vi "Construct Text Log Sink.vi"(7 "LogLevel":T1, 10 "File Name":string, 11 "Log File Folder":path) -> (3 "Text File Sink out":refnum<class "Text File Sink.lvclass">)   [LabVIEW 2018, in "MVA Framework.lvlib" / "Text File Sink.lvclass"]
doc: "Construct an instance of text log sink. If no file name is input, the file name will be 'Application Directory Name Event Log'. If no log file folder is input, the log file folder will be Public Application Data\\Application Directory Name Event Logs. \n - File extension used is .txt. \n - File will be rolled over at 1Mb.\n - File name will include a timestamp when that file was created.\nFor control over these default values, use the advanced constructor."
uses:
  Text File Sink.lvclass
  Composed Log/Log Sink/Log Sink.lvclass
  Configuration.ctl
  <vilib>/Utility/sysdir.llb/System Directory Type.ctl
  Composed Log/Types/Log Level.ctl
  Composed Log/Composed Log.lvlib
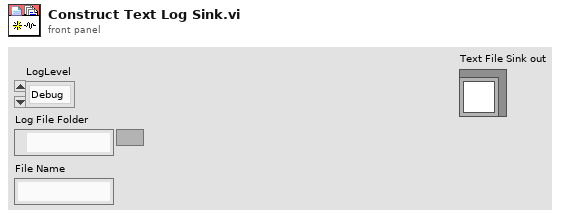
[diagram p1: front panel]
types:
  T1 = typedef "MVA Framework.lvlib/Composed Log.lvlib/Log Level.ctl" = enum16{"Debug", "Info", "Warning", "Error", "Critical"}
  T2 = typedef "MVA Framework.lvlib/Text File Sink.lvclass/Configuration.ctl" = cluster{"Folder":path, "Name":string, "Extension":string, "Max Size (MB)":i64, "Timestamp Filename":bool}
  T3 = typedef "System Directory Type.ctl" = i32
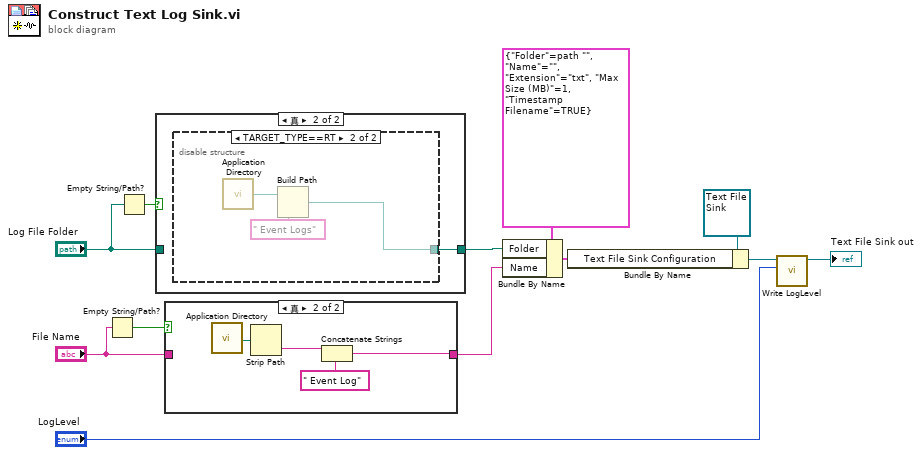
[diagram p0: block diagram]
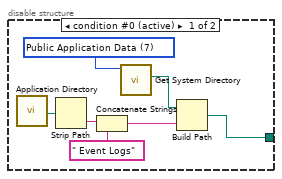
[diagram p4: hidden frame]
diagram:
  n1 = Empty String/Path?(string/path="File Name") -> (empty?=w4:bool)
  n2 = Empty String/Path?(string/path="Log File Folder") -> (empty?=w7:bool)
  n3 = case shown="真" w7 {
    tunnel: "Log File Folder" -> [w13 _]
    tunnel: [w13 w14] -> w5
    frame False {
    }
    frame True {
      n4 = disable-structure shown="TARGET_TYPE==RT" {
        disable-tunnel: [w15 w22] -> w14
        frame condition #0 (active) {
          w21 = T3 7 items=["User Home"=0, "User Desktop"=1, "User Documents"=2, "User Application Data"=3, "User Preferences"=4, "User Temporary"=5, "Public Documents"=6, "Public Application Data"=7, "Public Preferences"=8, "Public Cache"=13, "System Core Libraries"=9, "System Installed Libraries"=10, "Application Files"=11, "Boot Volume Root"=12] ("system directory type")
          n5 = call <vilib>:"Application Directory.vi"() -> ("Application Directory"=w20:path)
          n6 = Strip Path(path=w20) -> (name=w19:string)  [unwired: 1 out]
          n7 = Concatenate Strings(w19, " Event Logs" ("string")) -> (w17:string)
          n8 = call <vilib>:"Get System Directory.vi"("system directory type"=w21) -> ("system directory"=w16:path)  [unwired: 10 in]
          n9 = Build Path(base path=w16, name or relative path=w17) -> (appended path=w15:path)
        }
        frame condition #1 {
          n10 = call <vilib>:"Application Directory.vi"() -> ("Application Directory"=w23:path)
          n11 = Build Path(base path=w23, name or relative path=" Event Logs" ("string")) -> (appended path=w22:path)
        }
      }
    }
  }
  n12 = case shown="真" w4 {
    tunnel: "File Name" -> [w25 _]
    tunnel: [w25 w26] -> w2
    frame False {
    }
    frame True {
      n13 = call <vilib>:"Application Directory.vi"() -> ("Application Directory"=w29:path)
      n14 = Strip Path(path=w29) -> (name=w28:string)  [unwired: 1 out]
      n15 = Concatenate Strings(w28, " Event Log" ("string")) -> (w26:string)
    }
  }
  n16 = Bundle By Name(cluster=T2 {"Folder"=path "", "Name"="", "Extension"="txt", "Max Size (MB)"=1, "Timestamp Filename"=TRUE} ("Text File Sink Configuration"), "Folder"=w5, "Name"=w2) -> (w8:T2)
  n17 = Bundle By Name(cluster=refnum<class "Text File Sink.lvclass"> refnum ("Text File Sink in"), "Text File Sink Configuration"=w8) -> (w1:refnum<class "Text File Sink.lvclass">)
  n18 = call "Write LogLevel.vi"("LogLevel"="LogLevel", "Log Sink in"=w1) -> ("Log Sink out"=→"Text File Sink out":refnum<class "Text File Sink.lvclass">)  [unwired: 8 in, 1 out]
